vi "SetRingString.vi"(0 "Ring in":refnum<vi>, 1 "Priority(2)":u8=2, 2 "Severity(Critical)":string="Critical", 5 "RelativePathToINIFiles":string[](array[string]), 11 "ErrorArray In":errorcluster[](array[cluster])) -> (4 "IniFilePaths":path[](array[path]), 15 "ErrorArray Out out":errorcluster[](array[cluster]))   [LabVIEW 2018]
doc: "This VI sets the Text ring's values based on the type section in the configuration INI files."
uses:
  LV_Ini/Ini_lib.lvlib
  <userlib>/NIST/NISTErrorLib/NISTErrorLib.lvlib
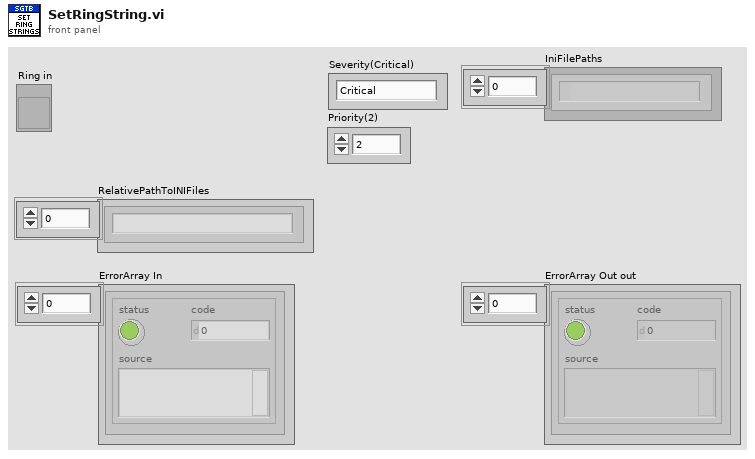
[diagram p1: front panel]
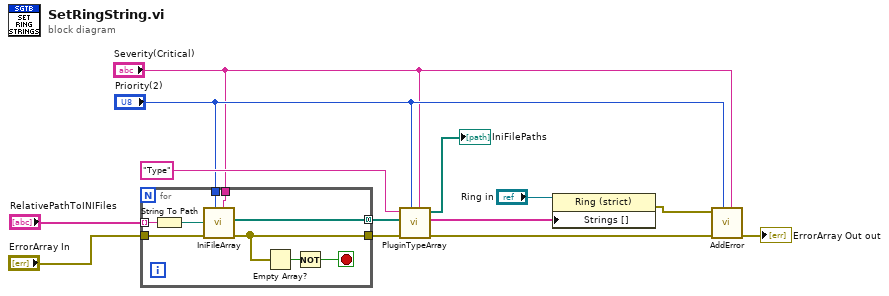
[diagram p0: block diagram]
diagram:
  n1 = for {
    tunnel: "RelativePathToINIFiles" -> [w22] mode=indexing
    tunnel: [w20] -> w11
    tunnel: [w19] -> w6 mode=concatenating
    tunnel: "ErrorArray In" -> [w18]
    tunnel: "Priority(2)" -> [w15]
    tunnel: "Severity(Critical)" -> [w14]
    stop <- w16 stop-if-true
    n2 = String To Path(string=w22) -> (path=w21:path)
    n3 = call "IniFileArray.vi"("Severity (Critical)"=w14, "Priority (2)"=w15, "ErrorArray In"=w18, "Relative Path to Plugins"=w21) -> ("ErrorArray Out"=w20:errorcluster[], "INIFilePaths"=w19:path[])  [unwired: 6 in]
    n4 = Empty Array?(array=w20) -> (empty?=w17:bool)
    n5 = Not(x=w17) -> (.not. x?=w16:bool)
  }
  n6 = call "PluginTypeArray.vi"("Severity (Critical)"="Severity(Critical)", "Priority (2)"="Priority(2)", "ErrorArray Out in"=w11, "INIFilePaths"=w6, "section"="Type") -> ("ErrorArray Out out"=w3:errorcluster[], "PluginTypes"=w5:string[], "IniFilePaths"=→"IniFilePaths":path[])  [unwired: 4 in]
  n7 = property class="Ring (strict)"(reference="Ring in", "Strings []"=w5) -> (error out=w7:errorcluster)  [unwired: 1 in, 1 out]
  n8 = call <userlib>:"AddError.vi"("Severity"="Severity(Critical)", "Priority"="Priority(2)", "ErrorArray"=w3, "error in (no error)"=w7) -> ("ErrorArray"=→"ErrorArray Out out":errorcluster[])  [unwired: 6 in, 1 out]
